vi "Periodic Tasks.vi"   [LabVIEW 2011]
doc: "This VI runs in parallel to other tasks. It can contain as many user-defined periodic loops as you need. These can carry out PID or other sorts of timed response."
uses:
  <vilib>/Platform/TimedLoop/XDataNode/timing_clust.ctl
  <vilib>/Platform/TimedLoop/XDataNode/nitl_modes.ctl
  <vilib>/Platform/TimedLoop/XDataNode/wakeup.ctl
  <vilib>/Rock Robotics/SystemInterfaces/Utilities/FPGA_UtilitiesLED State.ctl
  <vilib>/Rock Robotics/SystemInterfaces/Utilities/FPGA_UtilitiesLED Source.ctl
  Robot Global Data.vi
  <vilib>/Platform/TimedLoop/XDataNode/XDataNode.xnode
  <vilib>/Platform/TimedLoop/XDataNode/XDNodeRunTimeDep.lvlib
panel:
  # "Target Tracking"
types:
  T1 = typedef "XDNodeRunTimeDep.lvlib/timing_clust.ctl" = cluster{"Expected End [f-1]":u64, "Actual End [f-1]":u64, "Finished Late? [f-1]":bool, "Expected End [i-1]":u64, "Actual End [i-1]":u64, "Finished Late? [i-1]":bool, "Expected Start [i]":u64, "Actual Start [i]":u64, "Expected Start [f]":u64, "Actual Start [f]":u64, "Source Name":string, "Structure Name":string, "Period":i64, "Deadline":i64, "Offset":i64, "Start":i64, "Priority":i32, "Timeout":i32, "Mode":T2, "Wakeup Reason":T3, "Error":errorcluster, "Source Type":string, "Secondary Source Type":string, "Global End Time":u64, "Global Start Time":u64, "Frame Duration":u64, "Iteration Duration":u64, "Assigned CPU":i32, "I/O Scan Engine Mode":u32}
  T2 = typedef "XDNodeRunTimeDep.lvlib/nitl_modes.ctl" = enum32{"No Change", "Process missed periods, maintain original phase", "Discard missed periods, maintain original phase", "Process missed periods, ignore original phase", "Discard missed periods, ignore original phase"}
  T3 = typedef "XDNodeRunTimeDep.lvlib/wakeup.ctl" = enum32{"Normal", "Aborted", "Asynchronous wakeup", "Timing source error", "Timed loop error", "Timeout"}
  T4 = cluster{"Axis 1":dbl, "Axis 2":dbl, "Axis 3":dbl, "Axis 4":dbl, "Axis 5":dbl, "Axis 6":dbl, "Button 1":bool, "Button 2":bool, "Button 3":bool, "Button 4":bool, "Button 5":bool, "Button 6":bool, "Button 7":bool, "Button 8":bool, "Button 9":bool, "Button 10":bool, "Button 11":bool, "Button 12":bool}
  T5 = cluster{"Driver Station Digital Output (1-8)[0]":bool, "Driver Station Digital Output (1-8)[1]":bool, "Driver Station Digital Output (1-8)[2]":bool, "Driver Station Digital Output (1-8)[3]":bool, "Driver Station Digital Output (1-8)[4]":bool, "Driver Station Digital Output (1-8)[5]":bool, "Driver Station Digital Output (1-8)[6]":bool, "Driver Station Digital Output (1-8)[7]":bool, "Driver Station Digital Output (1-8)[8]":bool}
  T6 = typedef "FPGA_UtilitiesLED State.ctl" = enum16{"Off", "On", "Toggle"}
  T7 = typedef "FPGA_UtilitiesLED Source.ctl" = enum16{"User LED", "FPGA LED"}
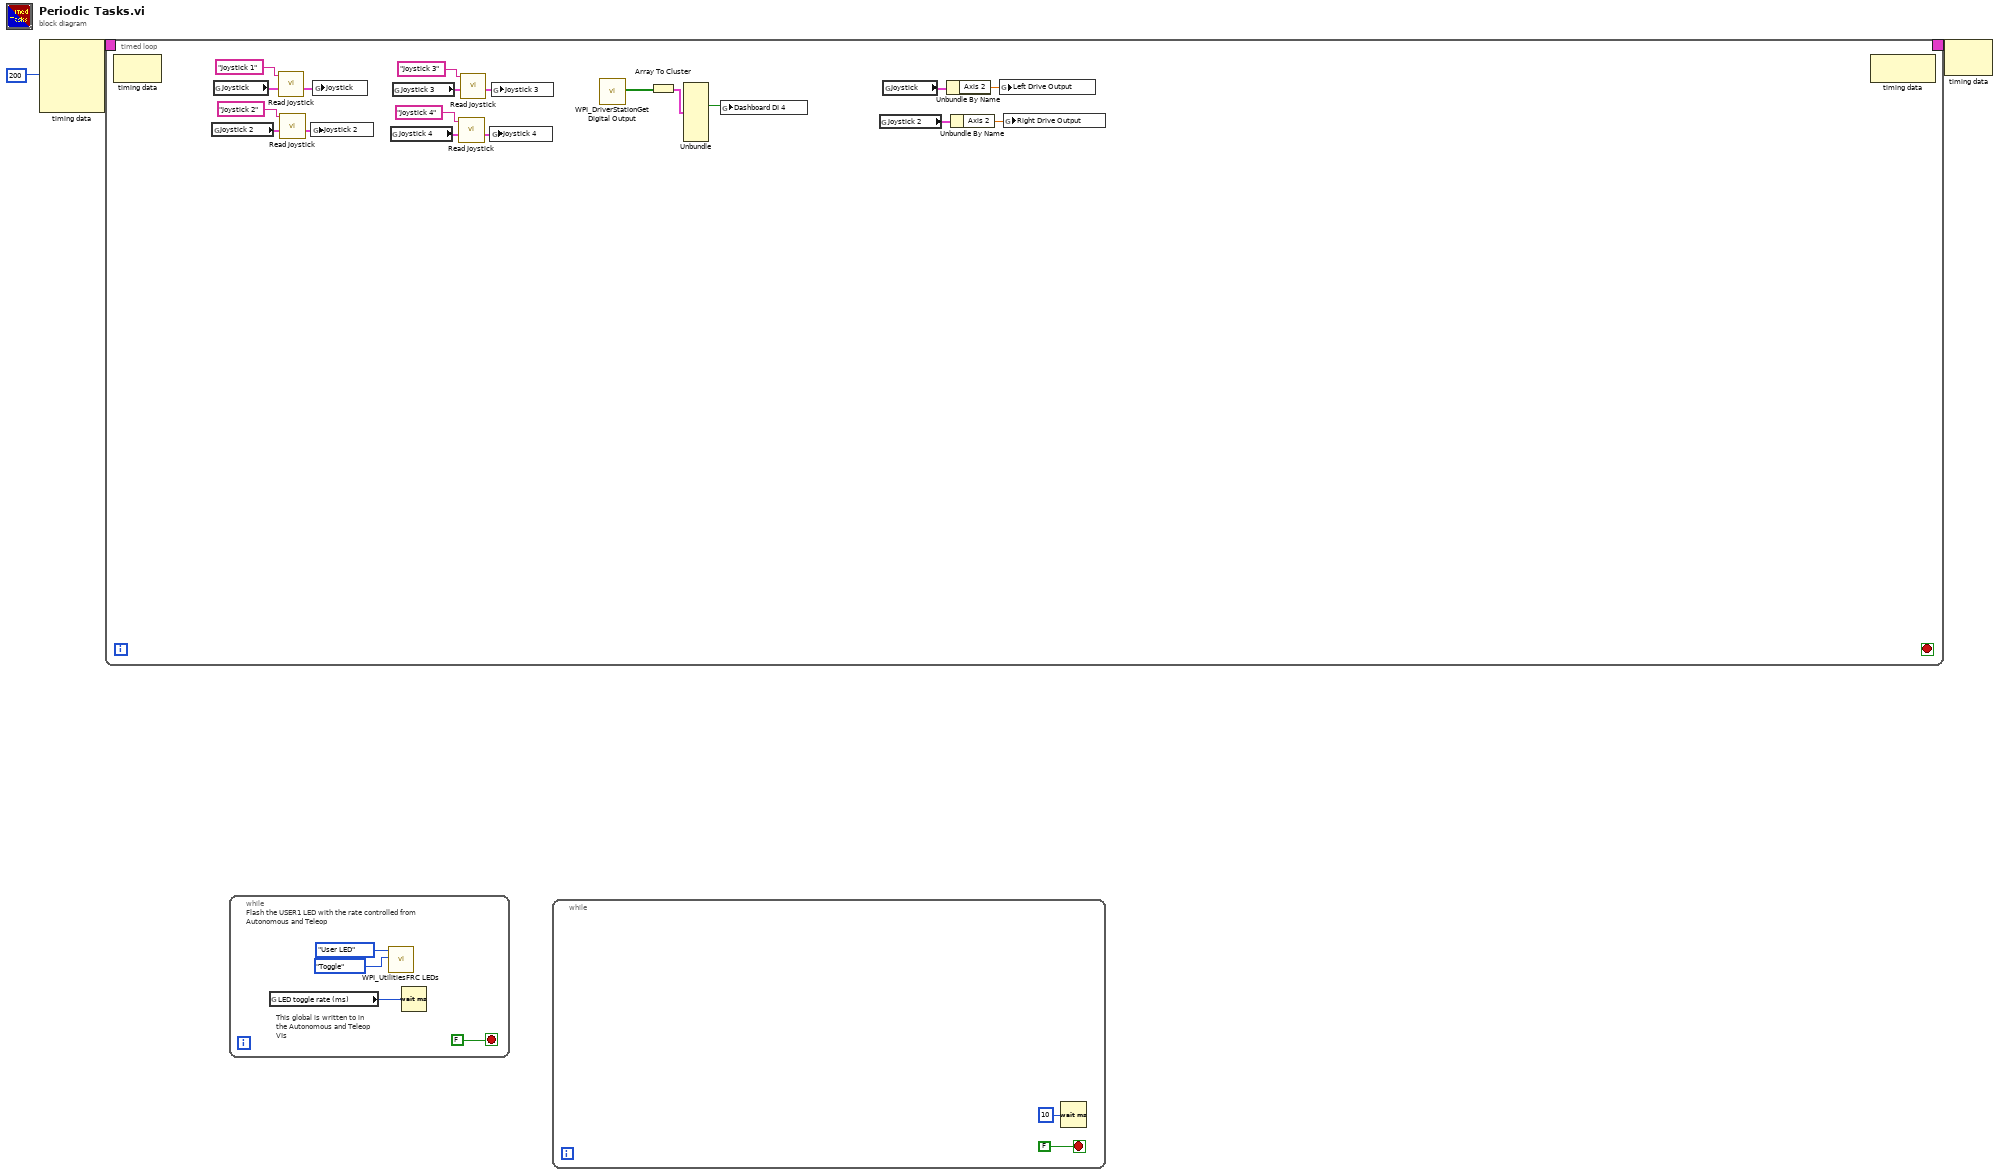
[diagram p0: block diagram]
diagram:
  n1 = node-c288(i64 200 ("Period")) -> (w3:T1)  [unwired: 3 in]
  n2 = timed-loop {
    timing: w3 -> [_]
    timing-out: [_] -> w2
    stop <- _ stop-if-true
    n3 = node-c288() -> ()  [unwired: 1 in, 1 out]
    n4 = global read "Robot Global Data.vi" "Joystick 2"() -> (w19:T4)
    n5 = global read "Robot Global Data.vi" "Joystick"() -> (w20:T4)
    n6 = call "Read Joystick.vi"("Joystick Input"=w20, "Joystick String"="Joystick 1") -> ("Joystick Output"=w22:T4)  [unwired: 9 in]
    n7 = call "Read Joystick.vi"("Joystick Input"=w19, "Joystick String"="Joystick 2") -> ("Joystick Output"=w17:T4)  [unwired: 9 in]
    n8 = global write "Robot Global Data.vi" "Joystick 2"(w17) -> ()
    n9 = global write "Robot Global Data.vi" "Joystick"(w22) -> ()
    n10 = global read "Robot Global Data.vi" "Joystick 4"() -> (w13:T4)
    n11 = global read "Robot Global Data.vi" "Joystick 3"() -> (w14:T4)
    n12 = call "Read Joystick.vi"("Joystick Input"=w13, "Joystick String"="Joystick 4") -> ("Joystick Output"=w11:T4)  [unwired: 9 in]
    n13 = call "Read Joystick.vi"("Joystick Input"=w14, "Joystick String"="Joystick 3") -> ("Joystick Output"=w16:T4)  [unwired: 9 in]
    n14 = global write "Robot Global Data.vi" "Joystick 4"(w11) -> ()
    n15 = global write "Robot Global Data.vi" "Joystick 3"(w16) -> ()
    n16 = call <vilib>:"WPI_DriverStationGet Digital Output.vi"() -> ("Driver Station Digital Output (1-8)"=w6:bool[])  [unwired: 10 in, 1 out]
    n17 = Array To Cluster(array=w6) -> (cluster=w5:T5)
    n18 = Unbundle(w5) -> ("Driver Station Digital Output (1-8)[3]"=w4:bool)  [unwired: 8 out]
    n19 = global write "Robot Global Data.vi" "Dashboard DI 4"(w4) -> ()
    n20 = global read "Robot Global Data.vi" "Joystick 2"() -> (w8:T4)
    n21 = global read "Robot Global Data.vi" "Joystick"() -> (w10:T4)
    n22 = Unbundle By Name(w10) -> ("Axis 2"=w9:dbl)
    n23 = Unbundle By Name(w8) -> ("Axis 2"=w7:dbl)
    n24 = global write "Robot Global Data.vi" "Left Drive Output"(w9) -> ()
    n25 = global write "Robot Global Data.vi" "Right Drive Output"(w7) -> ()
    n26 = node-c288() -> ()  [unwired: 1 in, 1 out]
  }
  n27 = while {
    stop <- FALSE stop-if-true
    # "This global is written to in the Autonomous and Teleop VIs"
    # "Flash the USER1 LED with the rate controlled from Autonomous and Teleop"
    n28 = global read "Robot Global Data.vi" "LED toggle rate (ms)"() -> (w25:u32)
    n29 = call <vilib>:"WPI_UtilitiesFRC LEDs.vi"("State"=FPGA_UtilitiesLED_State."Toggle", "LED Type"=FPGA_UtilitiesLED_Source."User LED") -> ()  [unwired: 1 in, 9 out]
    n30 = Wait (ms)(milliseconds to wait=w25) -> ()  [unwired: 1 out]
  }
  n31 = while {
    stop <- FALSE stop-if-true
    n32 = Wait (ms)(milliseconds to wait=u32 10) -> ()  [unwired: 1 out]
  }
  n33 = node-c288(w2) -> ()  [unwired: 1 out]
